vi "自动识别CAN卡.vi"(1 "设备索引号":u16(ring) items=["0", "1", "2", "3", "4", "5", "6", "7", "8", "9", "10", "11", "12", "13", "14", "15", ""], 2 "CAN端口":u16(ring) items=["0", "1"]) -> (14 "CAN卡类型 2":u32(ring)=4 items=["PCI5121"=1, "PCI9810"=2, "USBCAN1"=3, "USBCAN2"=4, "PCI9820"=5, "PCI5110"=7, "CANLite(mini)"=8, "ISA9620"=9, "ISA5420"=10, "PC104CAN"=11, "DNP9810"=13, "PCI9840B"=14, "PC104C2"=15, "PCI9820I"=16, "pec9920"=18, "USBCAN_E_U"=20, "USBCAN_2E_U"=21])   [LabVIEW 2013]
uses:
  data/ControlCAN.dll
panel:
  out "VCI_FILTER_RECORD":cluster{"ExtFrame":u32, "Start":u32, "End":u32}
  in  "e-u-baud":cluster{"数值":u32}
  in  "CAN卡类型":u32(ring)=4 items=["PCI5121"=1, "PCI9810"=2, "USBCAN1"=3, "USBCAN2"=4, "PCI9820"=5, "PCI5110"=7, "CANLite(mini)"=8, "ISA9620"=9, "ISA5420"=10, "PC104CAN"=11, "DNP9810"=13, "PCI9840B"=14, "PC104C2"=15, "PCI9820I"=16, "pec9920"=18, "USBCAN_E_U"=20, "USBCAN_2E_U"=21]
  in  "E-U_baud":u32(ring)=393223 items=["0x060003--1000Kbps"=393219, "0x060004--800Kbps"=393220, "0x060007--500Kbps"=393223, "0x1C0008--250Kbps"=1835016, "0x1C0011--125Kbps"=1835025, "0x160023--100Kbps"=1441827, "0x1C002C--50Kbps"=1835052, "0x1600B3--20Kbps"=1441971, "0x1C00E0--10Kbps"=1835232, "0x1C01C1--5Kbps"=1835457]
  in  "簇":T1={"打开CAN"=TRUE, "初始化CAN"=TRUE, "开始CAN"=TRUE, "重启"=TRUE, "关闭CAN"=TRUE}
  in  "VCI_INIT_CONFIG":T2={"AccCode"=0, "AccMask"=4294967295, "Reserved"=0, "Filter"=0, "Timing0"=191, "Timing1"=255, "Mode"=0}
  in  "error in (no error)":errorcluster caption="错误输入（无错误）"
  in  "操作类型":enum16{"初始化CAN", "关闭CAN"}(ring)
  out "CAN 操作结果":bool=TRUE
  in  "DeviceType 5":u16(ring)=1 items=["PCI5121"=1, "PCI9810"=2, "USBCAN1"=3, "USBCAN2"=4, "PCI9820"=5, "CAN232"=6, "PCI5110"=7, "CANLite(mini)"=8, "ISA9620"=9, "ISA5420"=10, "PC104CAN"=11, "CANETE"=12, "DNP9810"=13]
  in  "CAN Channel 3":u16(ring) items=["0", "1"]
  in  "DeviceType 4":u16(ring)=1 items=["PCI5121"=1, "PCI9810"=2, "USBCAN1"=3, "USBCAN2"=4, "PCI9820"=5, "CAN232"=6, "PCI5110"=7, "CANLite(mini)"=8, "ISA9620"=9, "ISA5420"=10, "PC104CAN"=11, "CANETE"=12, "DNP9810"=13]
  in  "Accept Code":u32 format="%08x"
  in  "Mask Code":u32=4294967295 format="%08x"
  in  "波特率":T3(ring)=enum."250Kbps"
  in  "工作方式":u8(ring) items=["Normal", "Listen Only"]
  in  "滤波方式":u8(ring)=1 items=["Dual Filter", "Single Filter"]
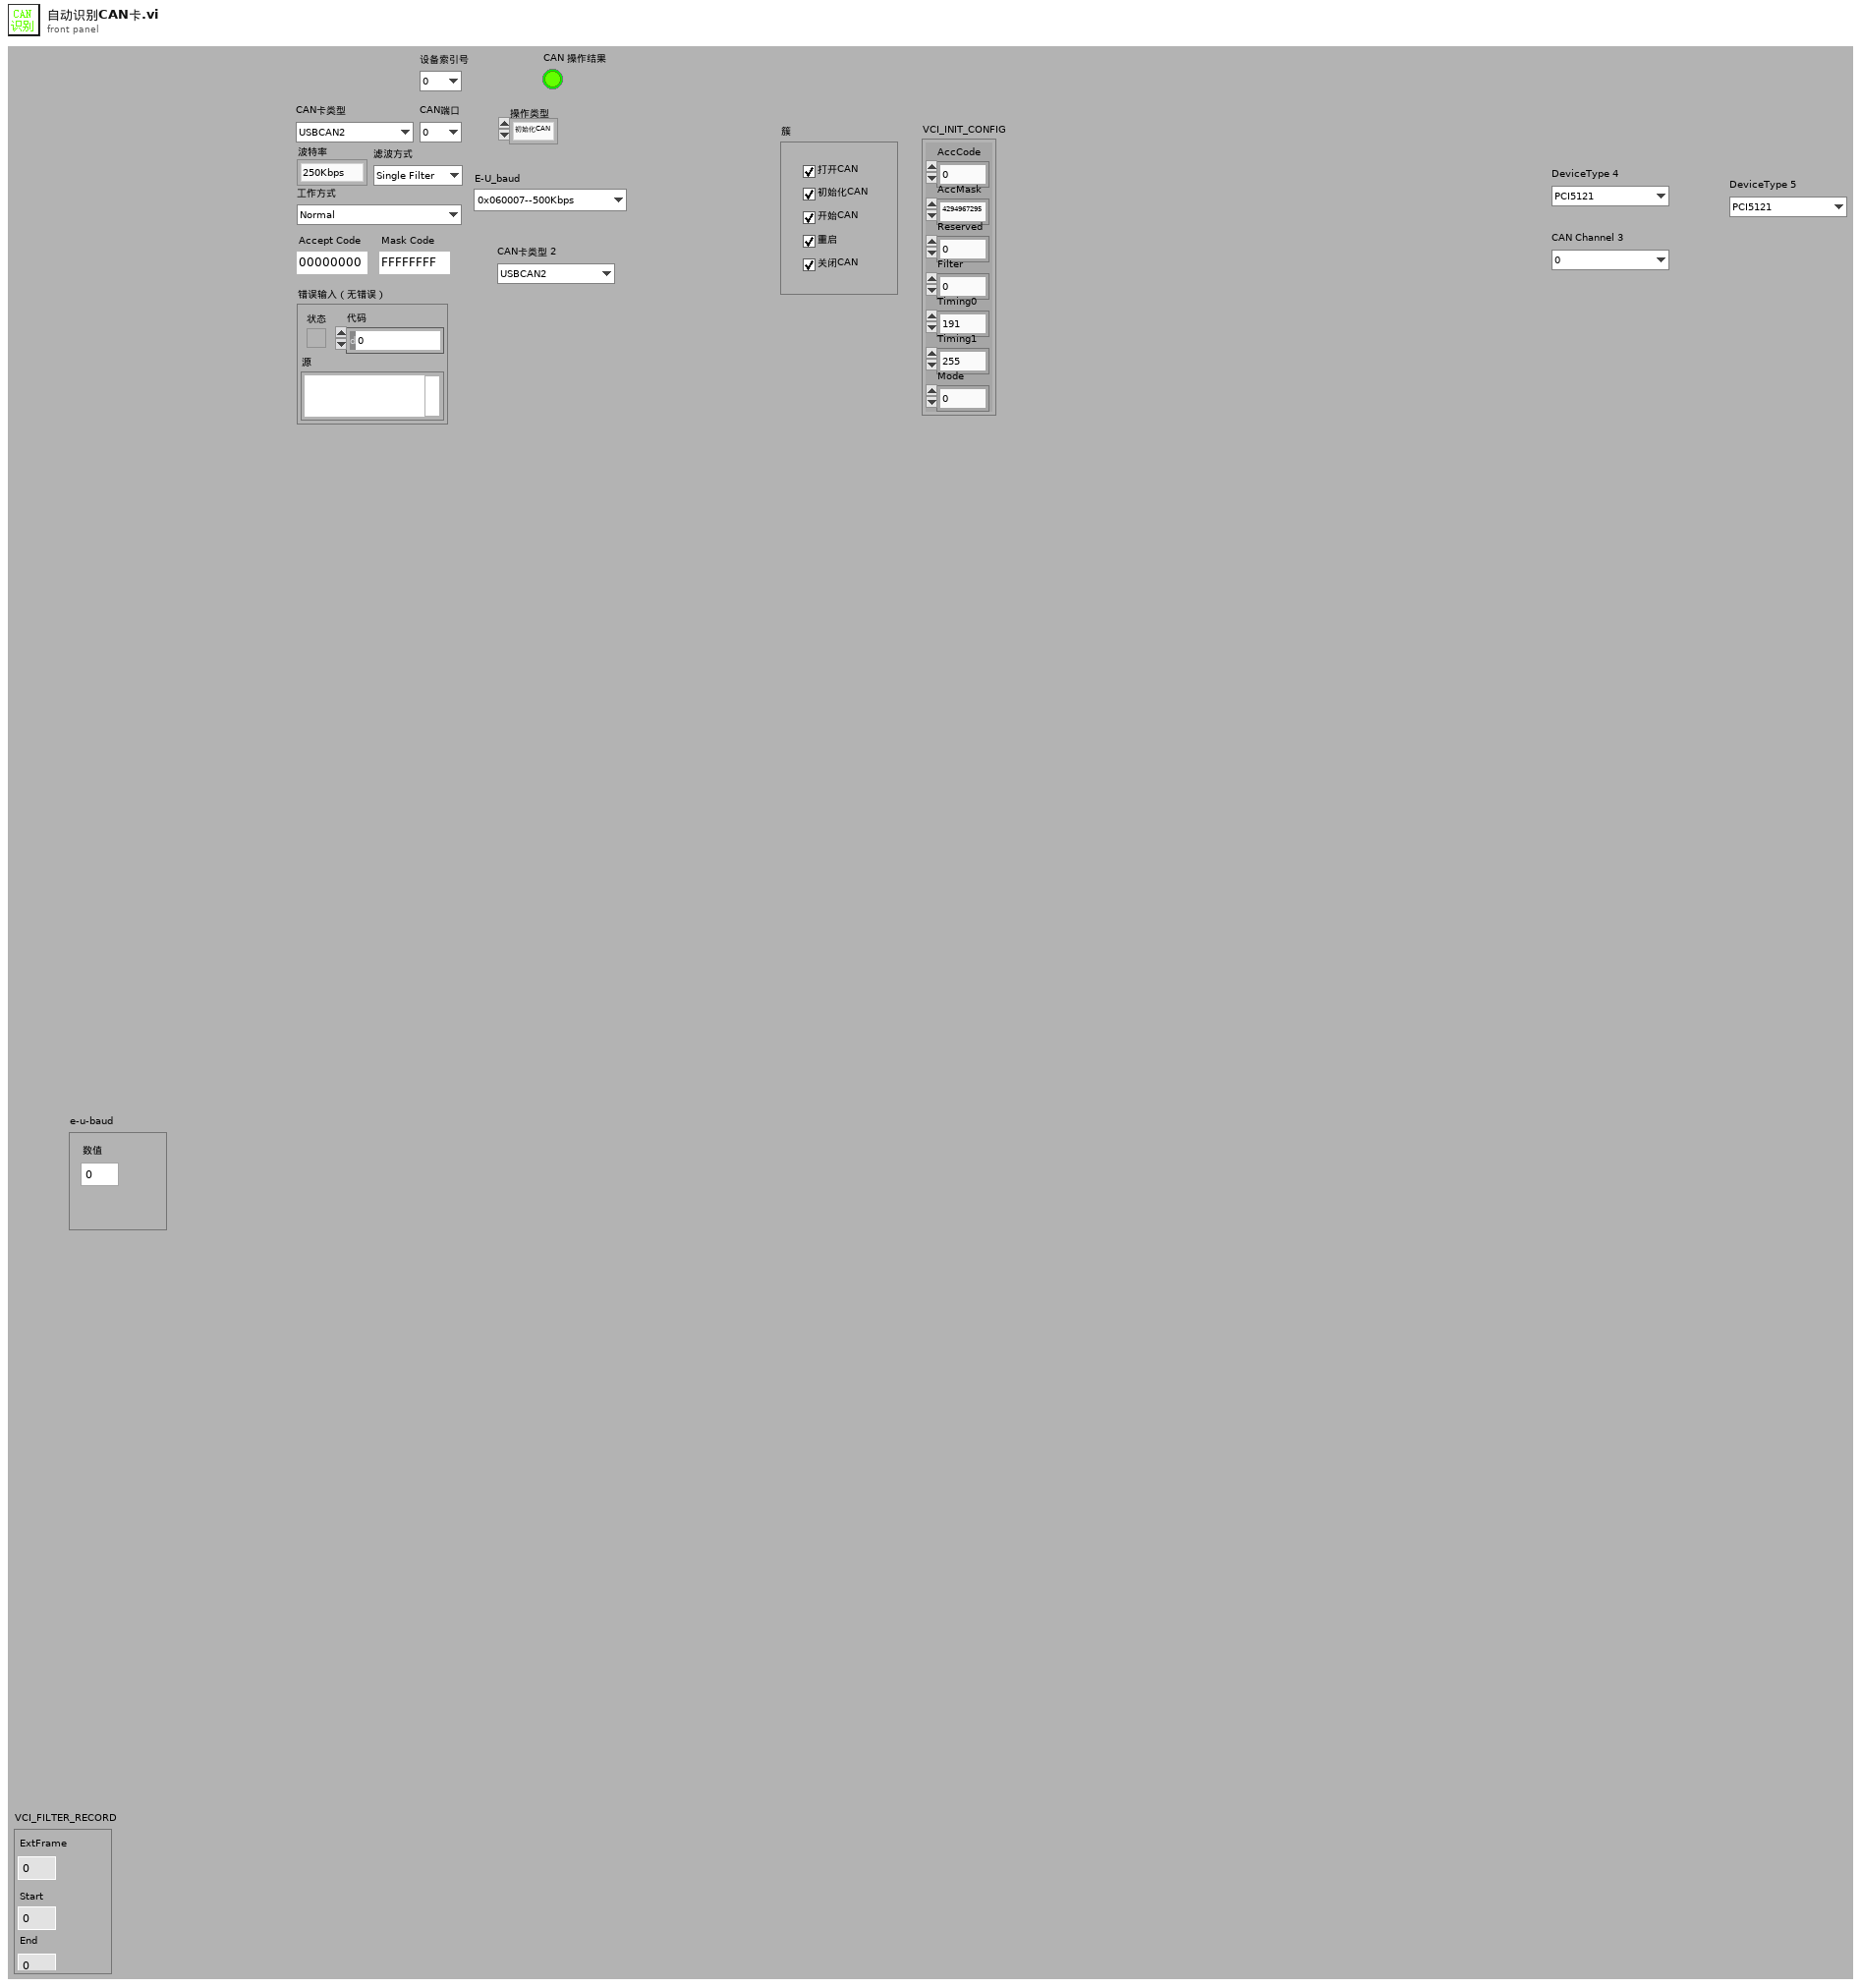
[diagram p1: front panel]
types:
  T1 = cluster{"打开CAN":bool, "初始化CAN":bool, "开始CAN":bool, "重启":bool, "关闭CAN":bool}
  T2 = cluster{"AccCode":u32, "AccMask":u32, "Reserved":u32, "Filter":u8, "Timing0":u8, "Timing1":u8, "Mode":u8}
  T3 = enum16{"5Kbps", "10Kbps", "20Kbps", "40Kbps", "50Kbps", "80Kbps", "100Kbps", "125Kbps", "200Kbps", "250Kbps", "400Kbps", "500Kbps", "666Kbps", "800Kbps", "1000Kbps"}
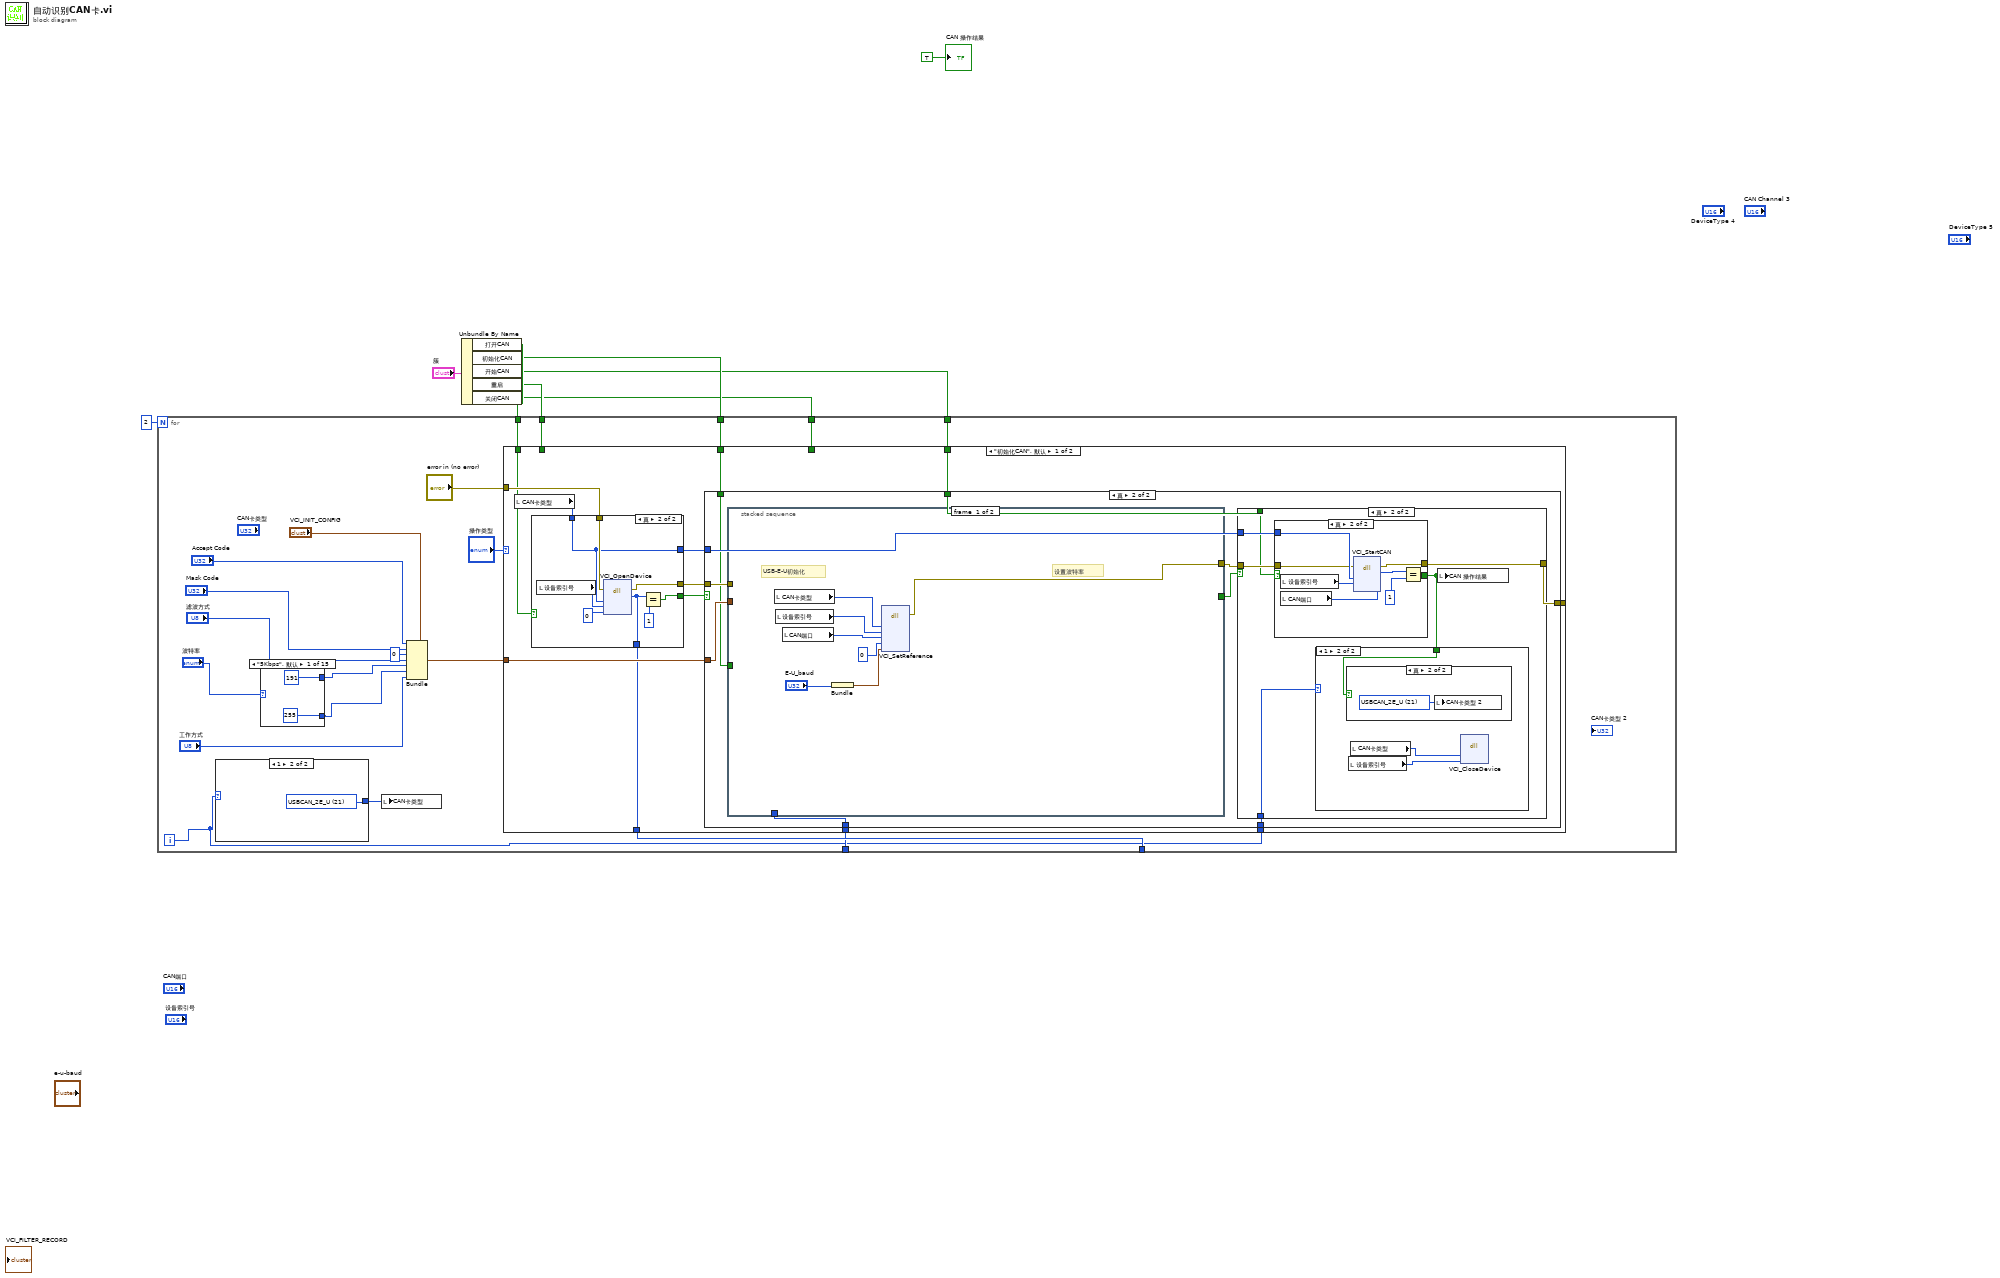
[diagram p0: block diagram]
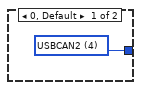
[diagram p2: hidden frame]
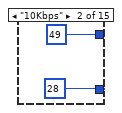
[diagram p3: hidden frame]
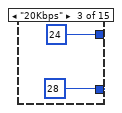
[diagram p4: hidden frame]
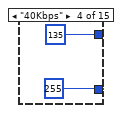
[diagram p5: hidden frame]
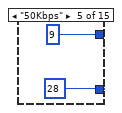
[diagram p6: hidden frame]
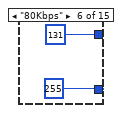
[diagram p7: hidden frame]
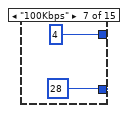
[diagram p8: hidden frame]
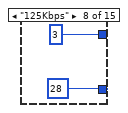
[diagram p9: hidden frame]
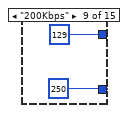
[diagram p10: hidden frame]
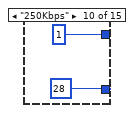
[diagram p11: hidden frame]
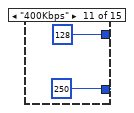
[diagram p12: hidden frame]
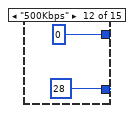
[diagram p13: hidden frame]
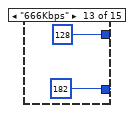
[diagram p14: hidden frame]
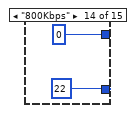
[diagram p15: hidden frame]
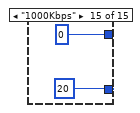
[diagram p16: hidden frame]
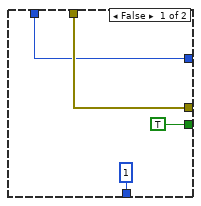
[diagram p17: hidden frame]
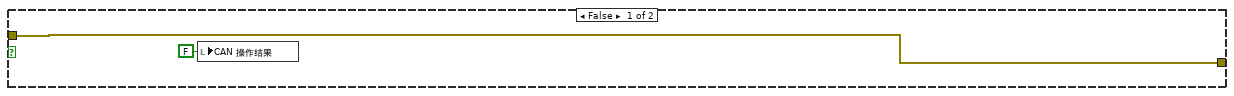
[diagram p18: hidden frame]
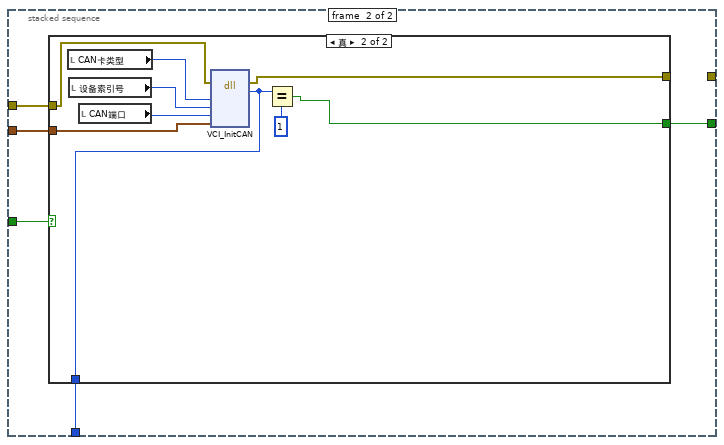
[diagram p19: hidden frame]
diagram:
  n1 = Unbundle By Name("簇") -> ("打开CAN"=w6:bool, "初始化CAN"=w5:bool, "开始CAN"=w4:bool, "重启"=w3:bool, "关闭CAN"=w2:bool)
  n2 = for {
    N: 2 -> [_]
    tunnel: [w17] -> _
    tunnel: [w16] -> _
    tunnel: w6 -> [w15]
    tunnel: w5 -> [w14]
    tunnel: w4 -> [w13]
    tunnel: w3 -> [w12]
    tunnel: w2 -> [w11]
    i -> [w9]
    n3 = case shown="1" w9 {
      tunnel: [w30 w31] -> w10
      frame 0, Default {
        w30 = u32 4 items=["PCI5121"=1, "PCI9810"=2, "USBCAN1"=3, "USBCAN2"=4, "PCI9820"=5, "PCI5110"=7, "CANLite(mini)"=8, "ISA9620"=9, "ISA5420"=10, "PC104CAN"=11, "DNP9810"=13, "PCI9840B"=14, "PC104C2"=15, "PCI9820I"=16, "pec9920"=18, "USBCAN_E_U"=20, "USBCAN_2E_U"=21] ("CAN卡类型")
      }
      frame 1 {
        w31 = u32 21 items=["PCI5121"=1, "PCI9810"=2, "USBCAN1"=3, "USBCAN2"=4, "PCI9820"=5, "PCI5110"=7, "CANLite(mini)"=8, "ISA9620"=9, "ISA5420"=10, "PC104CAN"=11, "DNP9810"=13, "PCI9840B"=14, "PC104C2"=15, "PCI9820I"=16, "pec9920"=18, "USBCAN_E_U"=20, "USBCAN_2E_U"=21] ("CAN卡类型")
      }
    }
    n4 = case shown="\"5Kbps\", 默认" "波特率" {
      tunnel: [191 49 24 135 9 131 4 3 129 1 128 0 128 0 0] -> w28
      tunnel: [255 28 28 255 28 255 28 28 250 28 250 28 182 22 20] -> w27
      frame "5Kbps", Default {
      }
      frame "10Kbps" {
      }
      frame "20Kbps" {
      }
      frame "40Kbps" {
      }
      frame "50Kbps" {
      }
      frame "80Kbps" {
      }
      frame "100Kbps" {
      }
      frame "125Kbps" {
      }
      frame "200Kbps" {
      }
      frame "250Kbps" {
      }
      frame "400Kbps" {
      }
      frame "500Kbps" {
      }
      frame "666Kbps" {
      }
      frame "800Kbps" {
      }
      frame "1000Kbps" {
      }
    }
    n5 = local write "CAN卡类型"(w10) -> ()
    n6 = Bundle(cluster="VCI_INIT_CONFIG", "AccCode"="Accept Code", "AccMask"="Mask Code", "Reserved"=u32 0, "Filter"="滤波方式", "Timing0"=w28, "Timing1"=w27, "Mode"="工作方式") -> (w23:T2)
    n7 = case shown="\"初始化CAN\", 默认" "操作类型" {
      tunnel: w23 -> [w72 _]
      tunnel: "error in (no error)" -> [w71 w151]
      tunnel: [w69 w149] -> _
      tunnel: [w68 _] -> w17
      tunnel: [w67 _] -> w16
      tunnel: w15 -> [w65 _]
      tunnel: w14 -> [w64 _]
      tunnel: w13 -> [w63 _]
      tunnel: w12 -> [_ w148]
      tunnel: w11 -> [_ w147]
      tunnel: w9 -> [w62 _]
      frame "初始化CAN", Default {
        n8 = local read "CAN卡类型"() -> (w66:u32)
        n9 = case shown="真" w65 {
          tunnel: [TRUE w83] -> w74
          tunnel: [w76 w79] -> w73
          tunnel: w71 -> [w78 w82]
          tunnel: [w78 w81] -> w70
          tunnel: [u32 1 ("返回类型") w80] -> w68
          tunnel: w66 -> [w76 w79]
          frame False {
          }
          frame True {
            n10 = local read "设备索引号"() -> (w84:u16)
            n11 = dll-call lib="PTH1labs FBluewave New EnergySVN_WorkBMS_Monitor_Bnet01trunkBMS_Monitor - 91版dataControlCAN.dll" fn="VCI_OpenDevice"(error in=w82, "DevType"=w79, "DevIndex"=w84, "Reserved"=0) -> (error out=w81:errorcluster, "返回类型"=w80:u32)  [unwired: 4 in, 2 out]
            n12 = Equal?(x=w80, y=u32 1) -> (x = y?=w83:bool)
          }
        }
        n13 = case shown="真" w74 {
          tunnel: w73 -> [_ w98]
          tunnel: w72 -> [_ w95]
          tunnel: w70 -> [w87 w93]
          tunnel: [w87 w97] -> w69
          tunnel: [_ w94] -> w67
          tunnel: w64 -> [_ w90]
          tunnel: w63 -> [_ w96]
          tunnel: w62 -> [_ w89]
          frame False {
            n14 = local write "CAN 操作结果"(FALSE ("初始化结果")) -> ()
          }
          frame True {
            n15 = stacked-sequence {
              tunnel: w95 -> [_ w110]
              tunnel: [_ w109] -> w94
              tunnel: w93 -> [_ w108]
              tunnel: [w99 _] -> w92
              tunnel: [_ w107] -> w91
              tunnel: w90 -> [_ w106]
              frame #0 {
                # "设置波特率"
                # "USB-E-U初始化"
                n16 = local read "CAN卡类型"() -> (w104:u32)
                n17 = local read "设备索引号"() -> (w103:u16)
                n18 = local read "CAN端口"() -> (w102:u16)
                n19 = Bundle("E-U_baud"="E-U_baud") -> (w100:cluster{"E-U_baud":u32})  [unwired: 1 in]
                n20 = dll-call lib="PTH1labs FBluewave New EnergySVN_WorkBMS_Monitor_Bnet01trunkBMS_Monitor - 91版dataControlCAN.dll" fn="VCI_SetReference"("DevType"=w104, "DevIndex"=w103, "CANInd"=w102, "RefType"=u32 0, "pData"=w100) -> (error out=w99:errorcluster)  [unwired: 5 in, 5 out]
              }
              frame #1 {
                n21 = case shown="真" w106 {
                  tunnel: w110 -> [_ w116]
                  tunnel: [_ w115] -> w109
                  tunnel: w108 -> [w111 w114]
                  tunnel: [w111 w113] -> _
                  tunnel: [_ w112] -> w107
                  frame False {
                  }
                  frame True {
                    n22 = local read "CAN卡类型"() -> (w119:u32)
                    n23 = local read "设备索引号"() -> (w118:u16)
                    n24 = local read "CAN端口"() -> (w117:u16)
                    n25 = dll-call lib="PTH1labs FBluewave New EnergySVN_WorkBMS_Monitor_Bnet01trunkBMS_Monitor - 91版dataControlCAN.dll" fn="VCI_InitCAN"(error in=w114, "DeviceType"=w119, "DeviceInd"=w118, "CANInd"=w117, "VCI_INIT_CONFIG"=w116) -> (error out=w113:errorcluster, w115:u32)  [unwired: 4 in, 3 out]
                    n26 = Equal?(x=w115, y=u32 1) -> (x = y?=w112:bool)
                  }
                }
              }
            }
            n27 = case shown="真" w91 {
              tunnel: w98 -> [_ w128]
              tunnel: w92 -> [w121 w127]
              tunnel: [w121 w126] -> w97
              tunnel: w96 -> [_ w125]
              tunnel: w89 -> [_ w124]
              frame False {
                n28 = local write "CAN 操作结果"(FALSE ("初始化结果")) -> ()
              }
              frame True {
                n29 = case shown="真" w125 {
                  tunnel: w128 -> [_ w144]
                  tunnel: [FALSE w141] -> w123
                  tunnel: w127 -> [w137 w140]
                  tunnel: [w137 w139] -> w126
                  frame False {
                  }
                  frame True {
                    n30 = local read "设备索引号"() -> (w143:u16)
                    n31 = local read "CAN端口"() -> (w142:u16)
                    n32 = dll-call lib="PTH1labs FBluewave New EnergySVN_WorkBMS_Monitor_Bnet01trunkBMS_Monitor - 91版dataControlCAN.dll" fn="VCI_StartCAN"(error in=w140, "DeviceType"=w144, "DeviceInd"=w143, "CANInd"=w142) -> (error out=w139:errorcluster, "返回类型"=w145:u32)  [unwired: 3 in, 3 out]
                    n33 = Equal?(x=w145, y=u32 1) -> (x = y?=w141:bool)
                  }
                }
                n34 = case shown="1" w124 {
                  tunnel: w123 -> [w131 w135]
                  frame 0, Default {
                    n35 = case shown="真" w131 {
                      frame False {
                      }
                      frame True {
                        w132 = u32 4 items=["PCI5121"=1, "PCI9810"=2, "USBCAN1"=3, "USBCAN2"=4, "PCI9820"=5, "PCI5110"=7, "CANLite(mini)"=8, "ISA9620"=9, "ISA5420"=10, "PC104CAN"=11, "DNP9810"=13, "PCI9840B"=14, "PC104C2"=15, "PCI9820I"=16, "pec9920"=18, "USBCAN_E_U"=20, "USBCAN_2E_U"=21] ("CAN卡类型 2")
                        n36 = local write "CAN卡类型 2"(w132) -> ()
                      }
                    }
                    n37 = local read "设备索引号"() -> (w129:u16)
                    n38 = local read "CAN卡类型"() -> (w130:u32)
                    n39 = dll-call lib="PTH1labs FBluewave New EnergySVN_WorkBMS_Monitor_Bnet01trunkBMS_Monitor - 91版dataControlCAN.dll" fn="VCI_CloseDevice"("DeviceType"=w130, "DeviceInd"=w129) -> ()  [unwired: 4 in, 4 out]
                  }
                  frame 1 {
                    n40 = case shown="真" w135 {
                      frame False {
                      }
                      frame True {
                        w136 = u32 21 items=["PCI5121"=1, "PCI9810"=2, "USBCAN1"=3, "USBCAN2"=4, "PCI9820"=5, "PCI5110"=7, "CANLite(mini)"=8, "ISA9620"=9, "ISA5420"=10, "PC104CAN"=11, "DNP9810"=13, "PCI9840B"=14, "PC104C2"=15, "PCI9820I"=16, "pec9920"=18, "USBCAN_E_U"=20, "USBCAN_2E_U"=21] ("CAN卡类型 2")
                        n41 = local write "CAN卡类型 2"(w136) -> ()
                      }
                    }
                    n42 = local read "设备索引号"() -> (w133:u16)
                    n43 = local read "CAN卡类型"() -> (w134:u32)
                    n44 = dll-call lib="PTH1labs FBluewave New EnergySVN_WorkBMS_Monitor_Bnet01trunkBMS_Monitor - 91版dataControlCAN.dll" fn="VCI_CloseDevice"("DeviceType"=w134, "DeviceInd"=w133) -> ()  [unwired: 4 in, 4 out]
                  }
                }
                n45 = local write "CAN 操作结果"(w123) -> ()
              }
            }
          }
        }
      }
      frame "关闭CAN" {
        n46 = case shown="真" w148 {
          tunnel: [TRUE w160] -> w152
          tunnel: w151 -> [w154 w156]
          tunnel: [w154 w155] -> w150
          frame False {
          }
          frame True {
            n47 = local read "设备索引号"() -> (w158:u16)
            n48 = local read "CAN端口"() -> (w157:u16)
            n49 = local read "CAN卡类型"() -> (w159:u32)
            n50 = dll-call lib="PTH1labs FBluewave New EnergySVN_WorkBMS_Monitor_Bnet01trunkBMS_Monitor - 91版dataControlCAN.dll" fn="VCI_ResetCAN"(error in=w156, "DeviceType"=w159, "DeviceInd"=w158, "CANInd"=w157) -> (error out=w155:errorcluster, "返回类型"=w161:u32)  [unwired: 3 in, 3 out]
            n51 = Equal?(x=w161, y=u32 1) -> (x = y?=w160:bool)
          }
        }
        n52 = case shown="真" w152 {
          tunnel: w150 -> [w163 w167]
          tunnel: [w163 w166] -> w149
          tunnel: w147 -> [_ w165]
          frame False {
            n53 = local write "CAN 操作结果"(FALSE ("CAN 操作结果")) -> ()
          }
          frame True {
            n54 = case shown="真" w165 {
              tunnel: [FALSE w173] -> w168
              tunnel: w167 -> [w169 w172]
              tunnel: [w169 w171] -> w166
              frame False {
              }
              frame True {
                n55 = local read "CAN卡类型"() -> (w175:u32)
                n56 = local read "设备索引号"() -> (w174:u16)
                n57 = dll-call lib="PTH1labs FBluewave New EnergySVN_WorkBMS_Monitor_Bnet01trunkBMS_Monitor - 91版dataControlCAN.dll" fn="VCI_CloseDevice"(error in=w172, "DeviceType"=w175, "DeviceInd"=w174) -> (error out=w171:errorcluster, "返回类型"=w176:u32)  [unwired: 3 in, 2 out]
                n58 = Equal?(x=w176, y=u32 1) -> (x = y?=w173:bool)
              }
            }
            n59 = local write "CAN 操作结果"(w168) -> ()
          }
        }
      }
    }
  }
  "CAN 操作结果" <- TRUE ("CAN 操作结果")
